vi "Remove Dead Enqueuers.vi"(8 "error in (no error)":errorcluster, 10 "Enqueuers to remove":string[](array[string]), 11 "Subsciptions in":T1[](array[typedef])) -> (0 "error out":errorcluster, 3 "Subsciptions out":T1[](array[typedef]))   [LabVIEW 2020, in "Publisher.lvlib" / "Publisher.lvclass"]
doc: "Remove dead enqueuers from 'Subscriptions in'"
uses:
  Publisher.lvclass
  Controls/Ctl_Subscription Element.ctl
  PPL/HDH.Actor Framework.Core.Actor.lvlibp/1abvi3w/vi.lib/ActorFramework/Message Enqueuer/Message Enqueuer.lvclass
  PPL/HDH.Actor Framework.Core.Utility.lvlibp
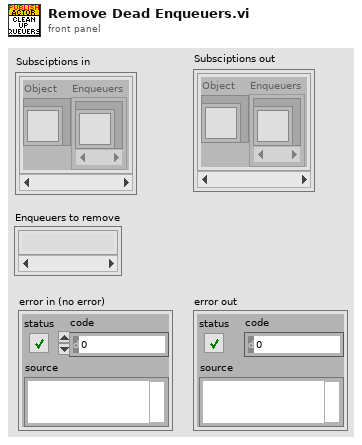
[diagram p1: front panel]
types:
  T1 = typedef "Publisher.lvlib/Publisher.lvclass/Ctl_Subscription Element.ctl" = cluster{"Object":refnum<class>, "Enqueuers":refnum<class "Message Enqueuer.lvclass">[]}
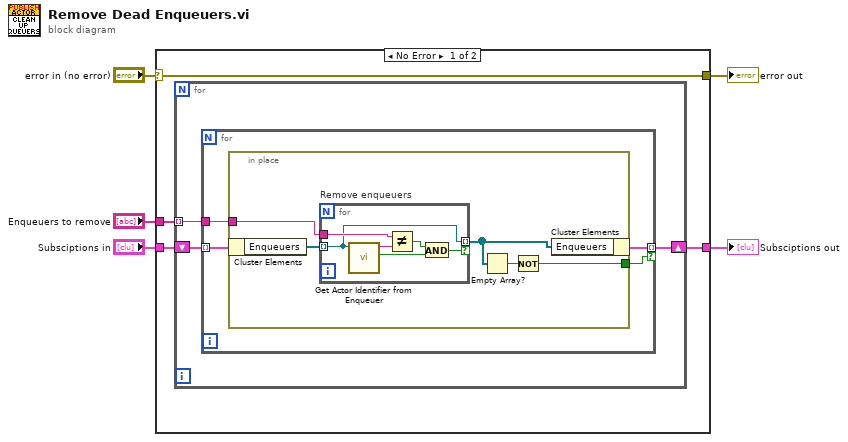
[diagram p0: block diagram]
diagram:
  n1 = case shown="No Error" "error in (no error)" {
    selector: "error in (no error)" -> [w6 w29]
    tunnel: "Subsciptions in" -> [w9 w28]
    tunnel: "Enqueuers to remove" -> [w8 _]
    tunnel: [w7 w28] -> w3
    tunnel: [w6 w29] -> w1
    frame No Error {
      n2 = for {
        tunnel: w8 -> [w11] mode=indexing
        shift-right: [w10] -> w7
        shift-left: w9 -> [w12]
        n3 = for {
          tunnel: w12 -> [w16] mode=indexing
          tunnel: w11 -> [w15]
          tunnel: [w14] -> w10 mode=indexing if=w13
          n4 = in-place {
            in-place-border: w15 -> [w20]
            in-place-border: [w17] -> w13
            n5 = in-place-cluster #1(w16) -> ("Enqueuers"=w21:refnum<class "Message Enqueuer.lvclass">[])
            n6 = for "Remove enqueuers" {
              tunnel: w21 -> [w23] mode=indexing
              tunnel: w20 -> [w27]
              tunnel: [w23] -> w19 mode=indexing if=w22
              n7 = call "Get Actor Identifier from Enqueuer.vi"("Message Enqueuer in"=w23) -> ("Valid Enqueuer?"=w24:bool, "Actor ID string out"=w26:string)  [unwired: 9 in]
              n8 = Not Equal?(x=w27, y=w26) -> (x != y?=w25:bool)
              n9 = And(x=w25, y=w24) -> (x .and. y?=w22:bool)
            }
            n10 = Empty Array?(array=w19) -> (empty?=w18:bool)
            n11 = Not(x=w18) -> (.not. x?=w17:bool)
            n12 = in-place-cluster #1("Enqueuers"=w19) -> (w14:T1)
          }
        }
      }
    }
    frame Error {
    }
  }
  "error out" <- w1
  "Subsciptions out" <- w3
